vi "Configure Trigger Model SMU Measure Action.vi"(0 "VISA resource name":refnum<visa-resource-name>, 1 "Reading Buffer 1 (smua.nvbuffer1)":string="smua.nvbuffer1", 2 "Reading Buffer 2 (smua.nvbuffer2)":string="smua.nvbuffer2", 5 "Source Measure Unit Channel (0: Channel A)":i32(ring) items=["Channel A", "Channel B"], 7 "Measurement Type (0: Current)":i32(ring) items=["Current", "Voltage", "Resistance", "Power", "Current and Voltage"], 9 "Measurement Action (0: Disable Measurement)":i32(ring) items=["Disable Measurement", "Enable Measurement", "Enable Asynchronous Measurement "], 11 "error in (no error)":errorcluster) -> (4 "VISA resource name out":refnum<visa-resource-name>, 15 "error out":errorcluster)   [LabVIEW 2019, in "Keithley 2600 Series.lvlib"]
doc: "Configures the measure action for the trigger model SMU (Source Measure Unit)."
uses:
  Keithley 2600 Series.lvlib
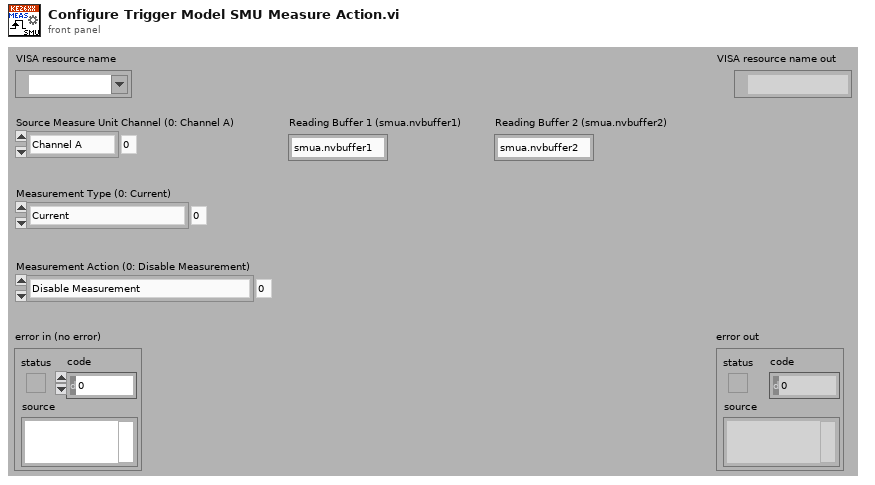
[diagram p1: front panel]
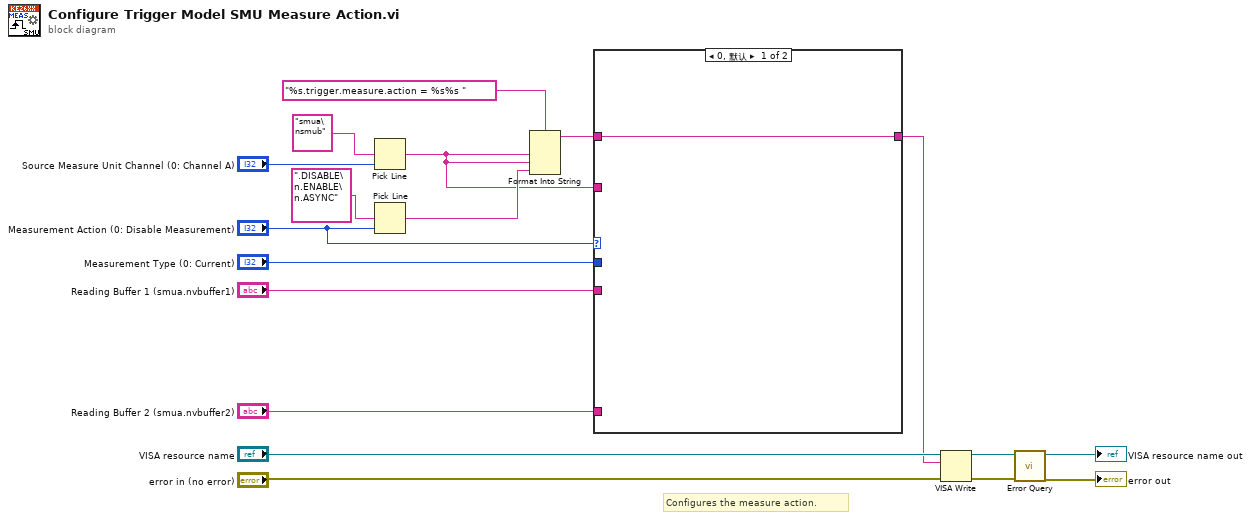
[diagram p0: block diagram]
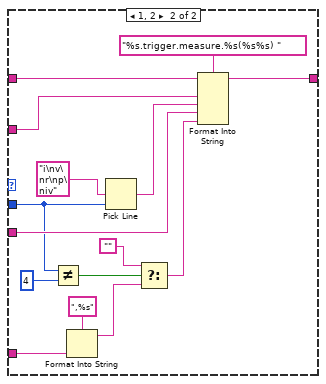
[diagram p2: hidden frame]
diagram:
  # "Configures the measure action."
  n1 = Pick Line(multi-line string="smua\nsmub", line index="Source Measure Unit Channel (0: Channel A)") -> (output string=w2:string)  [unwired: 1 in]
  n2 = Pick Line(multi-line string=".DISABLE\n.ENABLE\n.ASYNC", line index="Measurement Action (0: Disable Measurement)") -> (output string=w8:string)  [unwired: 1 in]
  n3 = Format Into String(format string="%s.trigger.measure.action = %s%s ", w2, w2, w8) -> (resulting string=w7:string)  [unwired: 2 in, 1 out]
  n4 = case shown="0, 默认" "Measurement Action (0: Disable Measurement)" {
    tunnel: w7 -> [w19 w20]
    tunnel: [w19 w30] -> w1
    tunnel: "Measurement Type (0: Current)" -> [_ w28]
    tunnel: w2 -> [_ w33]
    tunnel: "Reading Buffer 1 (smua.nvbuffer1)" -> [_ w29]
    tunnel: "Reading Buffer 2 (smua.nvbuffer2)" -> [_ w22]
    frame 0, Default {
    }
    frame 1, 2 {
      n5 = Not Equal?(x=w28, y=4) -> (x != y?=w26:bool)
      n6 = Format Into String(format string=",%s", w22) -> (resulting string=w21:string)  [unwired: 2 in, 1 out]
      n7 = Pick Line(multi-line string="i\nv\nr\np\niv", line index=w28) -> (output string=w31:string)  [unwired: 1 in]
      n8 = Select(t="", s=w26, f=w21) -> (s? t:f=w24:string)
      n9 = Format Into String(format string="%s.trigger.measure.%s(%s%s) ", initial string=w20, w33, w31, w29, w24) -> (resulting string=w30:string)  [unwired: 1 in, 1 out]
    }
  }
  n10 = VISA Write(VISA resource name="VISA resource name", write buffer=w1, error in (no error)="error in (no error)") -> (VISA resource name out=w15:refnum<visa-resource-name>, error out=w14:errorcluster)  [unwired: 1 out]
  n11 = call "Error Query.vi"("error in (no error)"=w14, "VISA resource name"=w15) -> ("error out"=→"error out":errorcluster, "VISA resource name out"=→"VISA resource name out":refnum<visa-resource-name>)  [unwired: 6 in, 2 out]
